vi "Valve-Open.vi"(7 "Device reference":refnum<vi>, 8 "error in (no error)":errorcluster, 9 "Eventstring":string="auto-generate") -> (0 "error out":errorcluster)   [LabVIEW 2015]
doc: "Opens a juicer valve.\n\nDevice reference: which valve?\nEventstring: used for timestamping\n--empty: no timestamp will be generated\n--unwired or \"auto-generate\": TS w/ default eventstring\n--otherwise: TS with user-provided string\n\nThe default eventstring is:\n[valve name].valve[valve #].open\nwhere [valve name] is the referenced juicer's front panel label text."
uses:
  Typedefs/Valve.ctl
  Rack/Typedefs/OutputRequest refnum.ctl
  Rack/Typedefs/OutputRequest.ctl
  Rack/Typedefs/InputData cluster.ctl
  Rack/Methods/Port drivers/DigitalInput-DataCluster.ctl
panel:
  # "(must be on same NI card)"
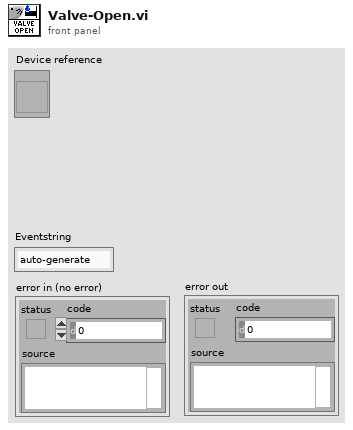
[diagram p1: front panel]
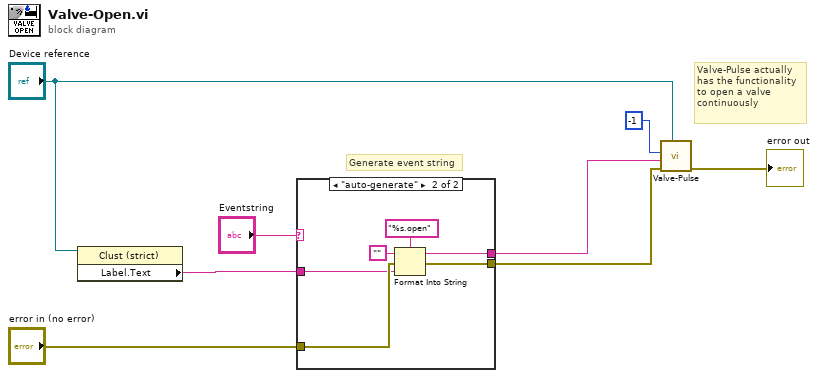
[diagram p0: block diagram]
diagram:
  # "Valve-Pulse actually\nhas the functionality\nto open a valve\ncontinuously"
  # "Generate event string"
  n1 = property class="Clust (strict)"(reference="Device reference") -> ("Label.Text"=w7:string)  [unwired: 1 in, 2 out]
  n2 = case shown="\"auto-generate\"" "Eventstring" {
    selector: "Eventstring" -> [w10 _]
    tunnel: w7 -> [_ w11]
    tunnel: [w10 w14] -> w4
    tunnel: "error in (no error)" -> [w9 w13]
    tunnel: [w9 w12] -> w2
    frame Default {
      # "Use user-provided string"
    }
    frame "auto-generate" {
      n3 = Format Into String(format string="%s.open", initial string="", error in=w13, w11) -> (resulting string=w14:string, error out=w12:errorcluster)
    }
  }
  n4 = call "Valve-Pulse.vi"("Device reference"="Device reference", "error in (no error)"=w2, "Eventstring"=w4, "Duration"=-1) -> ("error out"=→"error out":errorcluster)  [unwired: 6 in, 1 out]
